vi "Write log.vi"(8 "error in (no error)":errorcluster caption="에러 입력(에러 없음)", 10 "log":string, 11 "Script Line 입력":refnum<class "Script Line.lvclass">) -> (0 "error out":errorcluster caption="에러 출력", 3 "Script Line 출력":refnum<class "Script Line.lvclass">)   [LabVIEW 2020, in "Script Line.lvclass"]
uses:
  Script Line.lvclass
  Script Line.lvclass/Script Line.ctl
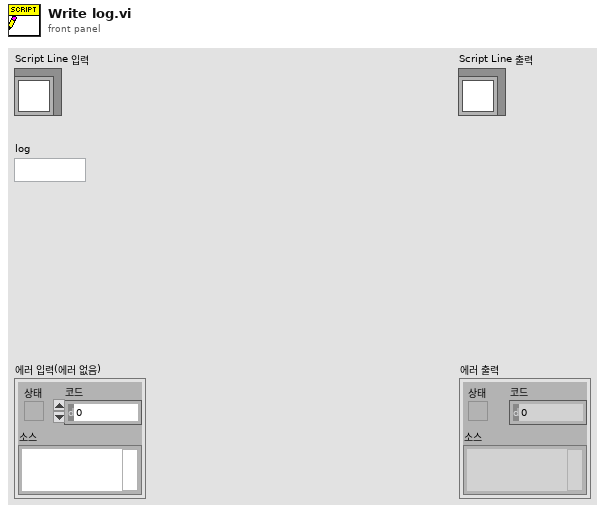
[diagram p1: front panel]
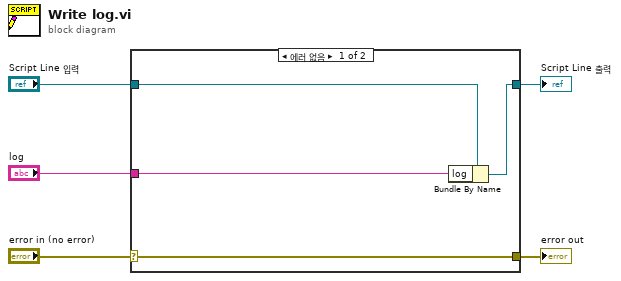
[diagram p0: block diagram]
diagram:
  n1 = case shown="에러 없음" "error in (no error)" {
    selector: "error in (no error)" -> [w9 w10]
    tunnel: [w9 w10] -> w4
    tunnel: [w7 w11] -> w2
    tunnel: "Script Line 입력" -> [w8 w11]
    tunnel: "log" -> [w6 _]
    frame No Error {
      n2 = Bundle By Name(cluster=w8, "log"=w6) -> (w7:refnum<class "Script Line.lvclass">)
    }
    frame Error {
    }
  }
  "error out" <- w4
  "Script Line 출력" <- w2
